vi "Script Name VI.vi"(8 "error in":errorcluster, 9 "Ref.Name VI":refnum<vi>, 10 "Conpane Map":T1(c390)) -> (0 "error out":errorcluster)   [LabVIEW 2020, in "_Msg Rescript.lvlib" / "_Msg Rescript.lvclass"]
uses:
  _Msg Rescript.lvclass
  <vilib>/Utility/traverseref.llb/TRef TravTarget.ctl
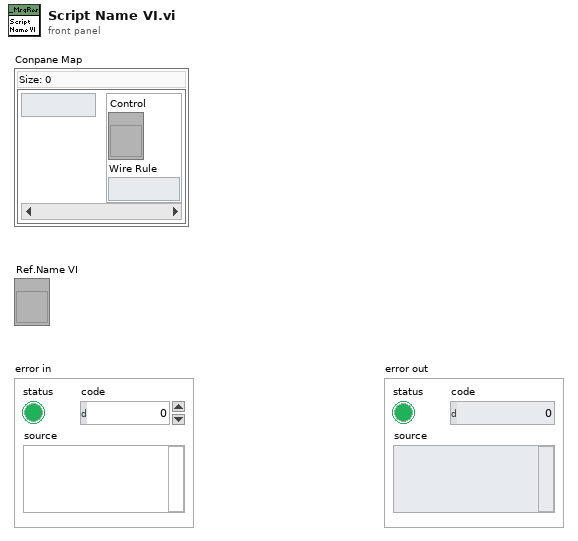
[diagram p1: front panel]
types:
  T1 = map{i32, cluster{"Control":refnum<vi>, "Wire Rule":enum16{"Invalid Wire Rule", "Required", "Recommended", "Optional", "Dynamic Dispatch"}}}
  T2 = typedef "TRef TravTarget.ctl" = enum16{"FP", "BD", "Other"}
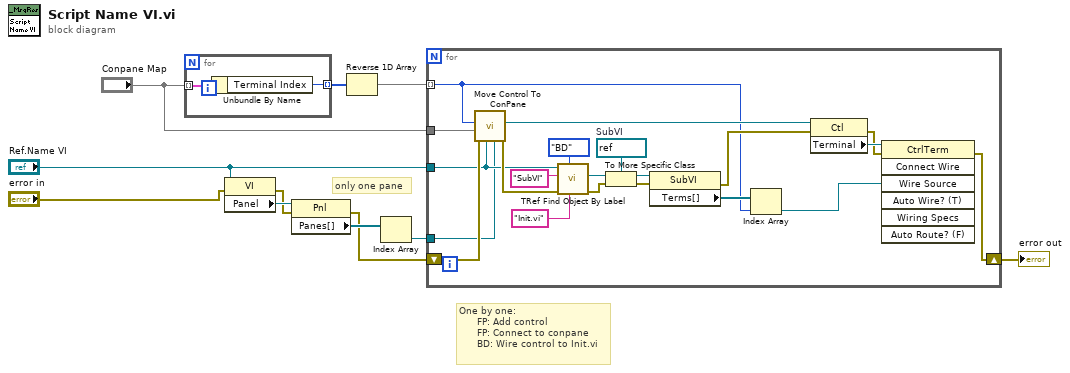
[diagram p0: block diagram]
diagram:
  # "only one pane"
  # "One by one:\n      FP: Add control\n      FP: Connect to conpane\n      BD: Wire control to Init.vi"
  n1 = for {
    tunnel: "Conpane Map" -> [w13] mode=indexing
    tunnel: [w12] -> w11 mode=indexing
    n2 = Unbundle By Name(w13) -> ("Terminal Index"=w12:i32)
  }
  n3 = property class="VI"(reference="Ref.Name VI", error in="error in") -> (error out=w7:errorcluster, "Panel"=w9:refnum<vi>)  [unwired: 1 out]
  n4 = property class="Pnl"(reference=w9, error in=w7) -> (error out=w6:errorcluster, "Panes[]"=w8:refnum<vi>[])  [unwired: 1 out]
  n5 = Reverse 1D Array(array=w11) -> (reversed array=w10:i32[])
  n6 = Index Array(array=w8) -> (element=w5:refnum<vi>)  [unwired: 1 in]
  n7 = for {
    tunnel: w10 -> [w14] mode=indexing
    tunnel: "Conpane Map" -> [w17]
    tunnel: w5 -> [w15]
    tunnel: "Ref.Name VI" -> [w16]
    shift-right: [w32] -> w1
    shift-left: w6 -> [w20]
    w30 = refnum<vi> refnum  # SubVI
    n8 = call "Move Control To ConPane.vi"("Pane"=w15, "Ref. VI"=w16, "error in"=w20, "Conpane Map"=w17, "Terminal Index"=w14) -> ("error out"=w19:errorcluster, "Control"=w18:refnum<vi>)  [unwired: 5 in]
    n9 = call <vilib>:"TRef Find Object By Label.vi"("Label"="Init.vi", "Traverse Target"=TRef_TravTarget."BD", "error in (no error)"=w19, "Class Name"="SubVI", "VI Ref"=w16) -> ("error out"=w29:errorcluster, "Found Obj Ref"=w24:refnum<vi>)  [unwired: 3 in, 2 out]
    n10 = To More Specific Class(target class=w30, reference=w24, error in=w29) -> (specific class reference=w27:refnum<vi>, error out=w26:errorcluster)
    n11 = property class="SubVI"(reference=w27, error in=w26) -> (error out=w21:errorcluster, "Terms[]"=w25:refnum<vi>[])  [unwired: 1 out]
    n12 = Index Array(array=w25, index=w14) -> (element=w22:refnum<vi>)
    n13 = property class="Ctl"(reference=w18, error in=w21) -> (error out=w33:errorcluster, "Terminal"=w34:refnum<vi>)  [unwired: 1 out]
    n14 = invoke class="CtrlTerm" method="Connect Wire"(reference=w34, error in=w33, "Wire Source"=w22) -> (error out=w32:errorcluster)  [unwired: 4 in, 6 out]
  }
  "error out" <- w1
